vi "LVFunction_Imop_GetExePathToConvertionTools.vi"(11 "error in (no error)":errorcluster) -> (4 "ExePath":path)   [LabVIEW 2018]
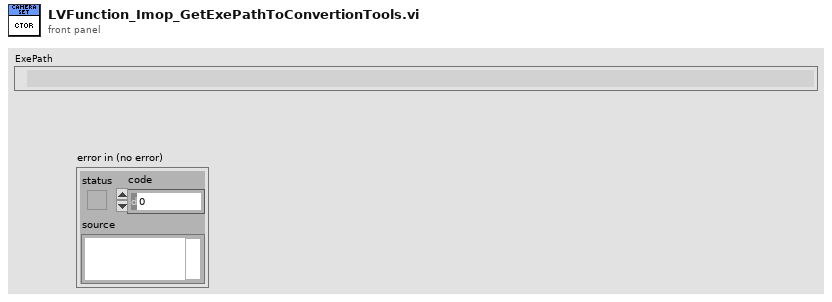
[diagram p1: front panel]
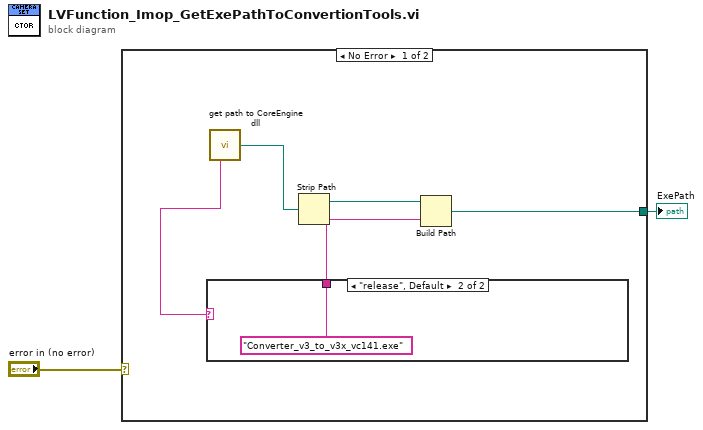
[diagram p0: block diagram]
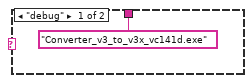
[diagram p2: hidden frame]
diagram:
  n1 = case shown="No Error" "error in (no error)" {
    tunnel: [w5 _] -> w1
    frame No Error {
      n2 = call "get path to CoreEngine dll.vi"() -> ("path to wavekit library"=w7:path, "Release/Debug"=w3:string)  [unwired: 14 in]
      n3 = case shown="\"release\", Default" w3 {
        tunnel: ["Converter_v3_to_v3x_vc141d.exe" ("name or relative path") "Converter_v3_to_v3x_vc141.exe" ("name or relative path")] -> w4
        frame "debug" {
        }
        frame "release", Default {
        }
      }
      n4 = Strip Path(path=w7) -> (stripped path=w6:path)  [unwired: 1 out]
      n5 = Build Path(base path=w6, name or relative path=w4) -> (appended path=w5:path)
    }
    frame Error {
    }
  }
  "ExePath" <- w1
